vi "Create Table.vi"() -> ()   [LabVIEW 2011]
panel:
  out "Picture Out":picture
  in  "Picture in":picture
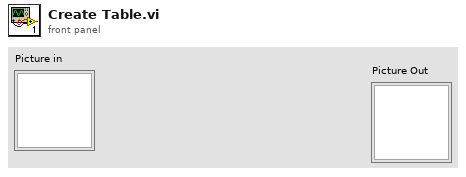
[diagram p1: front panel]
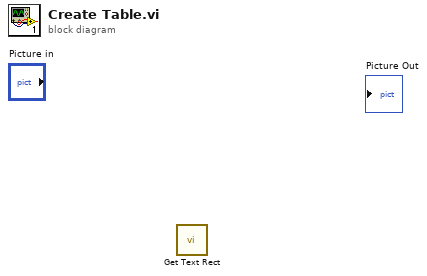
[diagram p0: block diagram]
diagram:
  n1 = call <vilib>:"Get Text Rect.vi"() -> ()  [unwired: 9 in, 1 out]
